vi "Delete Destination.vi"(8 "error in (no error)":errorcluster, 10 "Name":string, 11 "SigMan in":refnum<class "SignalManager.lvclass">) -> (0 "error out":errorcluster, 3 "SigMan out":refnum<class "SignalManager.lvclass">)   [LabVIEW 2015, in "SignalManager.lvclass"]
uses:
  SignalManager.lvclass
  SignalManager.lvclass/SignalManager.ctl
  Channel/Channel.lvclass/Channel.ctl
  Channel/Read Destination.vi
  Channel/Channel.lvclass
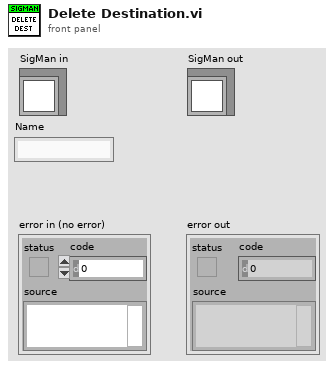
[diagram p1: front panel]
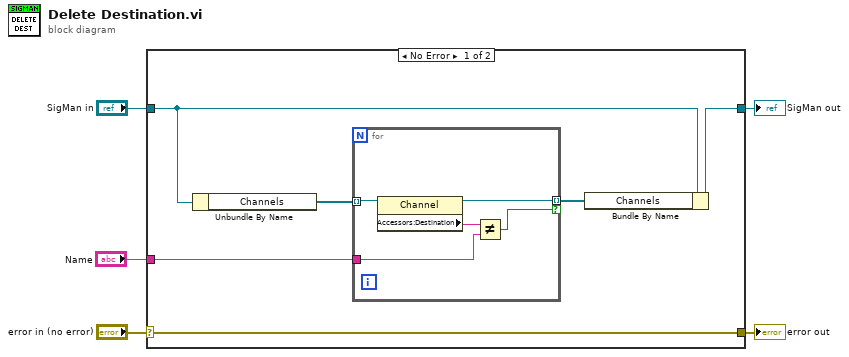
[diagram p0: block diagram]
diagram:
  n1 = case shown="No Error" "error in (no error)" {
    selector: "error in (no error)" -> [w11 w18]
    tunnel: [w11 w18] -> w4
    tunnel: [w7 w17] -> w2
    tunnel: "SigMan in" -> [w9 w17]
    tunnel: "Name" -> [w8 _]
    frame No Error {
      n2 = Unbundle By Name(w9) -> ("Channels"=w10:refnum<class "Channel.lvclass">[])
      n3 = for {
        tunnel: w10 -> [w16] mode=indexing
        tunnel: w8 -> [w14]
        tunnel: [w13] -> w6 mode=indexing if=w12
        n4 = property class="Channel"(reference=w16) -> (reference out=w13:refnum<class "Channel.lvclass">, "Accessors:Destination"=w15:string)  [unwired: 1 in, 1 out]
        n5 = Not Equal?(x=w15, y=w14) -> (x != y?=w12:bool)
      }
      n6 = Bundle By Name(cluster=w9, "Channels"=w6) -> (w7:refnum<class "SignalManager.lvclass">)
    }
    frame Error {
    }
  }
  "error out" <- w4
  "SigMan out" <- w2
